vi "WebBrowser.vi"(10 "File":path, 11 "ProjectRef":refnum<vi>) -> ()   [LabVIEW 2020, in "WebView2-Viewer.lvlib"]
uses:
  WebView2-Viewer.lvlib
  DP_WebView_class/DP_WebView.lvclass
  C:/Projects/DependencyViewer/DependencyViewer/DP_WebView_class/data/Microsoft.Web.WebView2.WinForms.dll
  DP_WebView_class/data/Microsoft.Web.WebView2.WinForms.dll
panel:
  in  "Webview container":refnum<k24>(container)
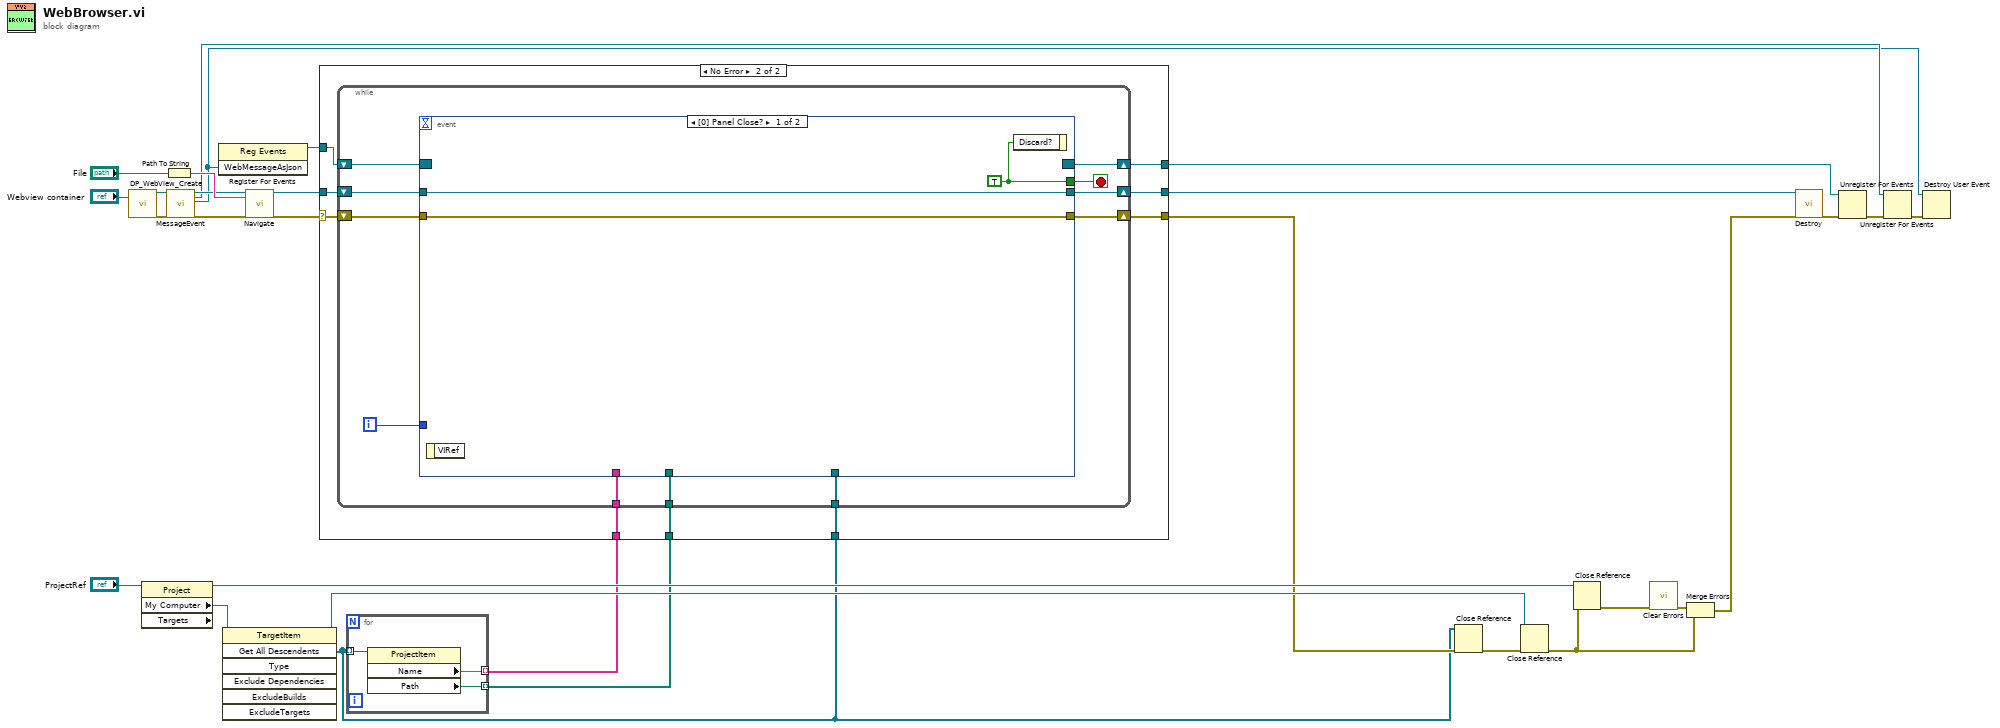
[diagram p0: block diagram]
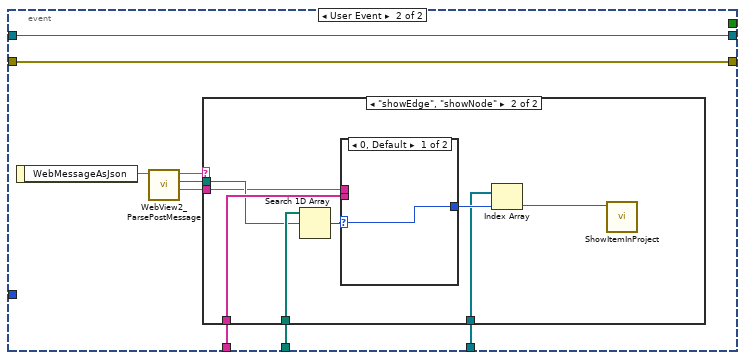
[diagram p3: hidden frame]
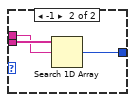
[diagram p5: hidden frame]
diagram:
  n1 = call "DP_WebView_Create.vi"("Webview container"="Webview container") -> ("reference out"=w24:refnum<class "DP_WebView.lvclass">, "Error Out"=w23:errorcluster)  [unwired: 11 in, 6 out]
  n2 = property class="Project" props=["My Computer", "Targets"](reference="ProjectRef") -> (reference out=w10:refnum<vi>, "My Computer"=w11:refnum<vi>)  [unwired: 1 in, 2 out]
  n3 = Path To String(path="File") -> (string=w25:string)
  n4 = call "MessageEvent.vi"("reference in"=w24, "error in (no error)"=w23) -> ("reference out"=w21:refnum<class "DP_WebView.lvclass">, "Event Callback"=w17:refnum<k27>, "WebMessageAsJson"=w14:refnum<user-event>, "error out"=w22:errorcluster)  [unwired: 14 in]
  n5 = register-events(w14) -> (reference out=w19:refnum<event-registration>)  [unwired: 2 in, 1 out]
  n6 = invoke class="TargetItem" method="Get All Descendents"(reference=w11) -> (reference out=w9:refnum<vi>, "All Descendents"=w4:refnum<vi>[])  [unwired: 6 in, 5 out]
  n7 = call-dynamic "Navigate.vi"("reference in"=w21, "URL"=w25, "Error In"=w22) -> ("reference out"=w30:refnum<class "DP_WebView.lvclass">, "Error Out"=w28:errorcluster)  [unwired: 14 in, 1 out]
  n8 = for {
    tunnel: w4 -> [w31] mode=indexing
    tunnel: [w33] -> w5 mode=indexing
    tunnel: [w32] -> w6 mode=indexing
    n9 = property class="ProjectItem"(reference=w31) -> ("Name"=w32:string, "Path"=w33:path)  [unwired: 1 in, 2 out]
  }
  n10 = case shown="No Error" w28 {
    selector: w28 -> [w36 w42]
    tunnel: w30 -> [w35 w45]
    tunnel: [w35 w44] -> w29
    tunnel: [w36 w43] -> w8
    tunnel: w19 -> [w34 w41]
    tunnel: [w34 w40] -> w18
    tunnel: w4 -> [_ w39]
    tunnel: w6 -> [_ w38]
    tunnel: w5 -> [_ w37]
    frame Error {
    }
    frame No Error {
      n11 = while {
        shift-right: [w55] -> w44
        shift-left: w45 -> [w56]
        shift-right: [w54] -> w43
        shift-left: w42 -> [w53]
        shift-right: [w51] -> w40
        shift-left: w41 -> [w52]
        tunnel: w39 -> [w48]
        tunnel: w38 -> [w47]
        tunnel: w37 -> [w46]
        i -> [w49]
        stop <- w50 stop-if-true
        n12 = event shown="[0] Panel Close?" {
          selector: w52 -> [_ _]
          dyn-events: [_ _] -> w51
          timeout: _ -> [_ _]
          tunnel: w56 -> [w59 w68]
          tunnel: [w59 w68] -> w55
          tunnel: w53 -> [w58 w67]
          tunnel: [w58 w67] -> w54
          tunnel: [w57 _] -> w50
          tunnel: w49 -> [_ _]
          tunnel: w48 -> [_ w64]
          tunnel: w47 -> [_ w63]
          tunnel: w46 -> [_ w62]
          event Panel Close? {
            w57 = TRUE ("Discard?")
            n13 = event-data() -> ()  [unwired: 1 in, 1 out]
            n14 = event-data("Discard?"=w57) -> ()  [unwired: 1 in, 1 out]
          }
          event User Event {
            n15 = event-data() -> ("WebMessageAsJson"=w66:string)  [unwired: 1 in]
            n16 = call "WebView2_ParsePostMessage.vi"("WebMessageAsJson"=w66) -> ("ItemName"=w60:string, "ItemVI"=w61:path, "Action"=w65:string)  [unwired: 8 in]
            n17 = case shown="\"showEdge\", \"showNode\"" w65 {
              tunnel: w64 -> [_ w73]
              tunnel: w63 -> [_ w72]
              tunnel: w62 -> [_ w71]
              tunnel: w61 -> [_ w70]
              tunnel: w60 -> [_ w69]
              frame "False", Default {
              }
              frame "showEdge", "showNode" {
                n18 = Search 1D Array(1D array=w71, element=w70) -> (index of element=w74:i32)  [unwired: 1 in]
                n19 = case shown="0, Default" w74 {
                  selector: w74 -> [w77 _]
                  tunnel: w72 -> [_ w80]
                  tunnel: [w77 w79] -> w75
                  tunnel: w69 -> [_ w78]
                  frame 0, Default {
                  }
                  frame -1 {
                    n20 = Search 1D Array(1D array=w80, element=w78) -> (index of element=w79:i32)  [unwired: 1 in]
                  }
                }
                n21 = Index Array(array=w73, index=w75) -> (element=w76:refnum<vi>)
                n22 = call "ShowItemInProject.vi"("ProjectItem in"=w76) -> ()  [unwired: 10 in, 1 out]
              }
            }
          }
        }
      }
    }
  }
  n23 = Close Reference(reference=w4, error in (no error)=w8) -> (error out=w12:errorcluster)
  n24 = Close Reference(reference=w9, error in (no error)=w12) -> (error out=w1:errorcluster)
  n25 = Close Reference(reference=w10, error in (no error)=w1) -> (error out=w7:errorcluster)
  n26 = call <vilib>:"Clear Errors.vi"("error in (no error)"=w7) -> ("error out"=w3:errorcluster)  [unwired: 5 in, 1 out]
  n27 = Merge Errors(w3, w1) -> (w2:errorcluster)
  n28 = call-dynamic "Destroy.vi"("reference in"=w29, "Error In"=w2) -> ("Error Out"=w20:errorcluster)  [unwired: 16 in, 1 out]
  n29 = Unregister For Events(event registration refnum=w18, error in=w20) -> (error out=w16:errorcluster)
  n30 = Unregister For Events(event registration refnum=w17, error in=w16) -> (error out=w15:errorcluster)
  n31 = Destroy User Event(user event=w14, error in=w15) -> ()  [unwired: 1 out]
